vi "KeySwitched.vi"(8 "error in (no error)":errorcluster, 9 "Key":T1 {"Time" format="%<%.3X>T"}, 11 "Gviewer in":refnum<class "Gviewer.lvclass">) -> (0 "error out":errorcluster, 3 "Gviewer out":refnum<class "Gviewer.lvclass">, 5 "Char":i16)   [LabVIEW 2020, in "Sgraph_lib_V1.lvlib" / "Gviewer.lvclass"]
doc: "Andre Koelewijn, 8 jan 2021\n\nIf a switch is pressed then this VI hold the code for the action.\nIf a key stroke combined with another action is used then it is possible that such code resides in another part of the program."
uses:
  Gviewer.lvclass
  controls/KeyPress.ctl
  <vilib>/event_ctls.llb/eventvkey.ctl
  Gviewer.lvclass/Gviewer.ctl
  Common/controls/ToolTypeEnum.ctl
  Builds/Sgraph_lib_V1.lvlib
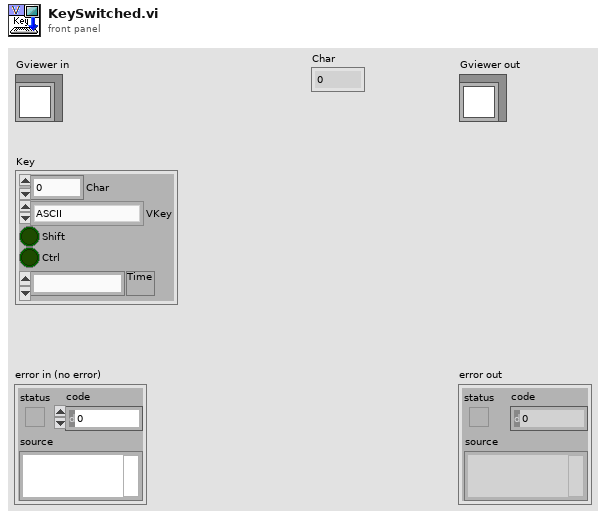
[diagram p1: front panel]
types:
  T1 = typedef "Sgraph_lib_V1.lvlib/Gviewer.lvclass/KeyPress.ctl" = cluster{"Char":i16, "VKey":T2, "Shift":bool, "Ctrl":bool, "Time":timestamp}
  T2 = typedef "eventvkey.ctl" = enum16{"ASCII", "Enter", "Return", "Shift", "Ctrl", "Alt", "Cmd", "Opt", "Caps", "NumLock", "Clear", "Break", "Up", "Down", "Left", "Right", "Insert", "Delete", "Home", "End", "PageUp", "PageDown", "Escape", "Help", "Pause", "ScrollLock", "F1", "F2", "F3", "F4", "F5", "F6", "F7", "F8", "F9", "F10", "F11", "F12", "F13", "F14", "F15", "F16", "F17", "F18", "F19", "F20", "F21", "F22", "F23", "F24", "Play", "VolumeUp", "VolumeDown", "Mute", "Two Byte Char"}
  T3 = typedef "Sgraph_lib_V1.lvlib/ToolTypeEnum.ctl" = enum16{"00_Esc button", "01_Undo", "02_HelpButton", "03_CursorViewButton", "04_AutoScale_Fit", "05_AutoScale_Stacked", "06_ZoomWindowStart", "07_ZoomTimeStart", "08_ZoomAmplitudeStart", "09", "10", "11", "12", "13", "14", "15", "16", "17", "18", "19", "20_VerticalScroll", "21_VerticalMove", "22_TimeScroll", "23_TimeMove", "24", "25", "26_ZoomWindowSize", "27_ZoomTimeWindowSize", "28_ZoomAmplitudeWindowSize", "29", "30_LegendMovePoint", "31_LegendMoveDrag", "32", "33", "34", "35", "36", "37", "38", "39", "40_AddYscalePoint", "41_AddYscalePlace", "42_AddYscaleMovePoint", "43_AddYscaleMoveDrag", "44_AddYscaleDeletePoint"}
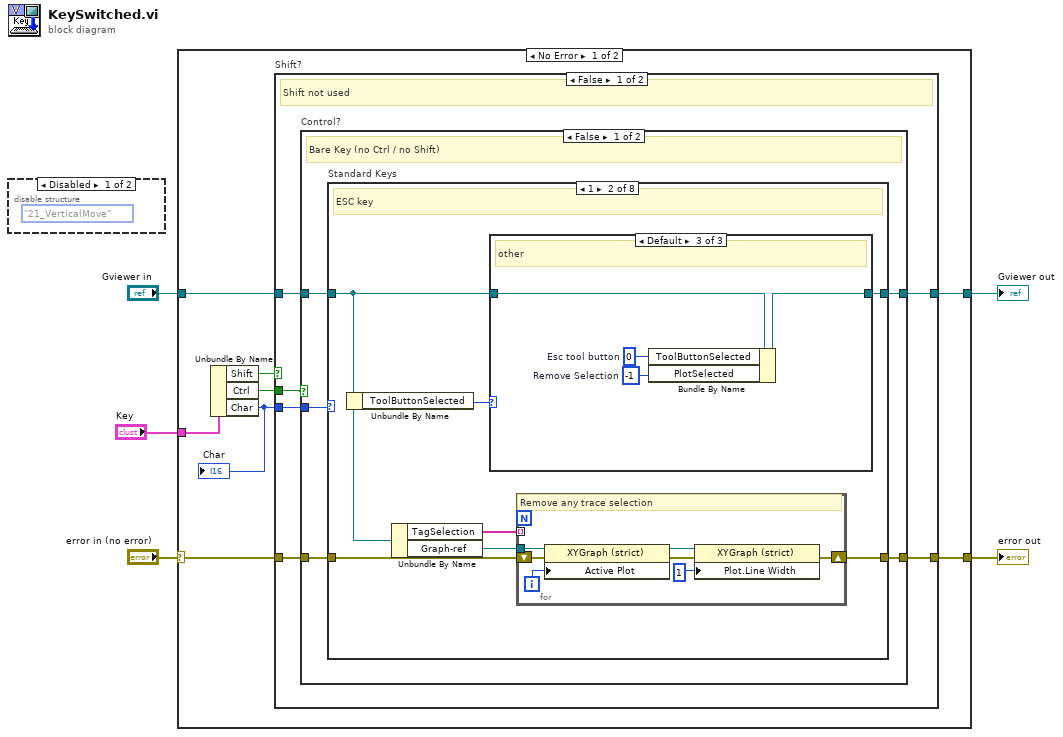
[diagram p0: block diagram]
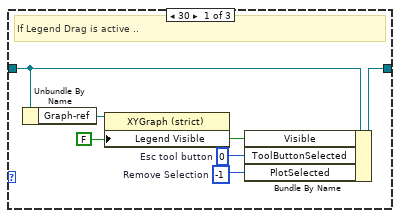
[diagram p4: hidden frame]
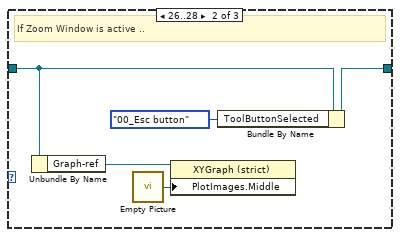
[diagram p5: hidden frame]
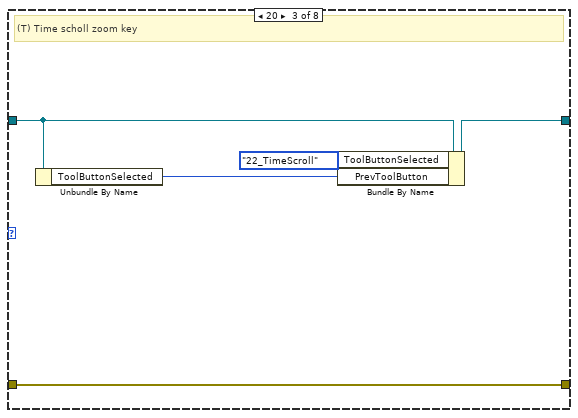
[diagram p6: hidden frame]
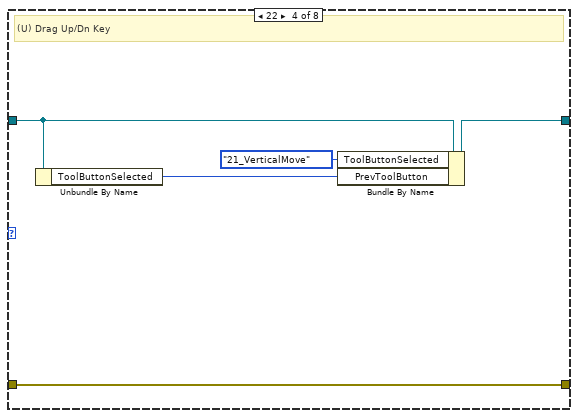
[diagram p7: hidden frame]
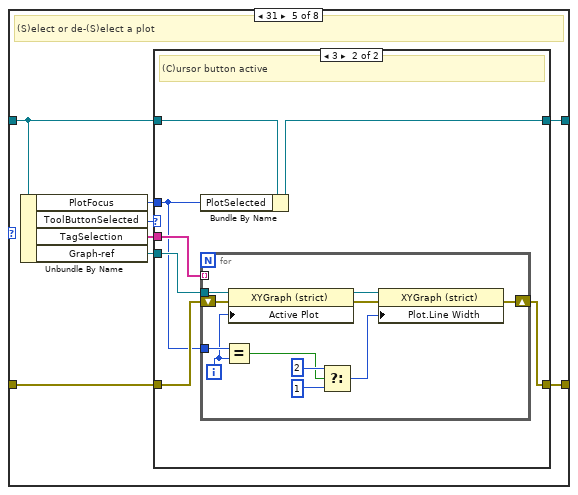
[diagram p8: hidden frame]
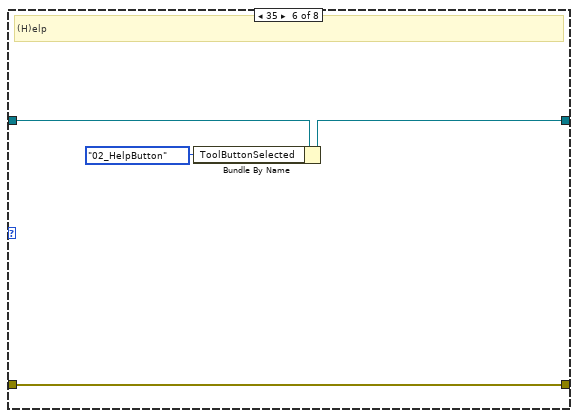
[diagram p10: hidden frame]
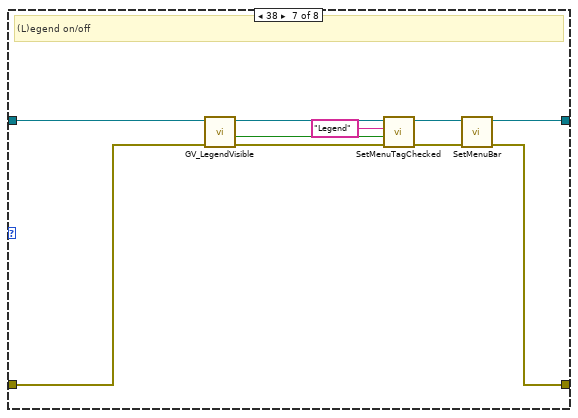
[diagram p11: hidden frame]
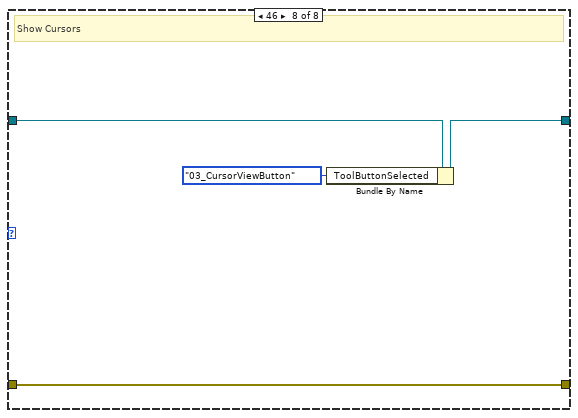
[diagram p12: hidden frame]
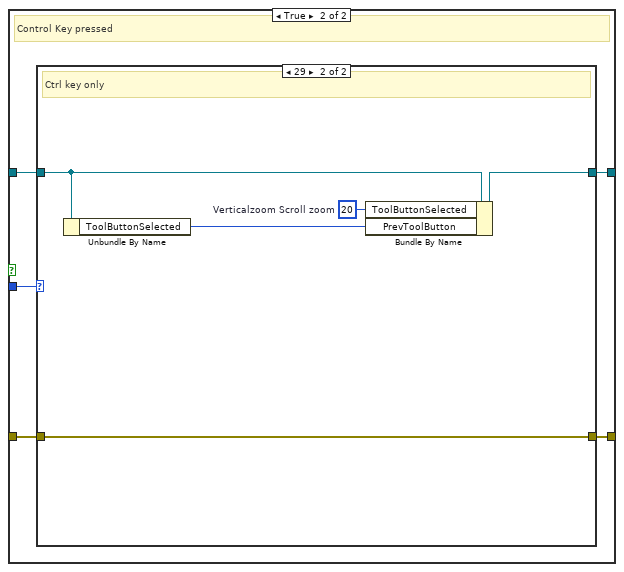
[diagram p13: hidden frame]
diagram:
  n1 = disable-structure shown="Disabled" {
    frame Disabled {
      (unwired) ToolTypeEnum."21_VerticalMove" ("Enum")
    }
    frame Enabled {
    }
  }
  n2 = case shown="No Error" "error in (no error)" {
    selector: "error in (no error)" -> [w8 w134]
    tunnel: [w7 w134] -> w4
    tunnel: [w9 w133] -> w2
    tunnel: "Gviewer in" -> [w10 w133]
    tunnel: "Key" -> [w13 _]
    frame No Error {
      n3 = Unbundle By Name(w13) -> ("Shift"=w12:bool, "Ctrl"=w11:bool, "Char"=w6:i16)
      "Char" <- w6
      n4 = case "Shift?" shown="False" w12 {
        tunnel: w11 -> [w19 w128]
        tunnel: w10 -> [w18 w127]
        tunnel: [w17 w126] -> w9
        tunnel: w8 -> [w16 w125]
        tunnel: [w15 w124] -> w7
        tunnel: w6 -> [w14 _]
        frame False {
          # "Shift not used"
          n5 = case "Control?" shown="False" w19 {
            tunnel: [w22 w114] -> w17
            tunnel: w18 -> [w23 w115]
            tunnel: [w20 w112] -> w15
            tunnel: w16 -> [w21 w113]
            tunnel: w14 -> [w24 w116]
            frame False {
              # "Bare Key (no Ctrl / no Shift)"
              n6 = case "Standard Keys" shown="1" w24 {
                tunnel: w23 -> [w26 w28 w59 w64 w70 w95 w101 w109]
                tunnel: [w26 w33 w58 w63 w69 w96 w104 w110] -> w22
                tunnel: [w25 w30 w57 w62 w72 w97 w103 w111] -> w20
                tunnel: w21 -> [w25 w29 w57 w62 w73 w97 w100 w111]
                frame Default {
                  # "Not implemented"
                }
                frame 1 {
                  # "ESC key"
                  n7 = Unbundle By Name(w28) -> ("ToolButtonSelected"=w27:i32)
                  n8 = Unbundle By Name(w28) -> ("TagSelection"=w32:string[], "Graph-ref"=w31:refnum<vi>)
                  n9 = case shown="Default" w27 {
                    tunnel: [w39 w44 w47] -> w33
                    tunnel: w28 -> [w36 w43 w45]
                    frame 30 {
                      w34 = -1  # Remove Selection
                      w35 = 0  # Esc tool button
                      w37 = FALSE
                      # "If Legend Drag is active .."
                      n10 = Unbundle By Name(w36) -> ("Graph-ref"=w38:refnum<vi>)
                      n11 = property class="XYGraph (strict)"(reference=w38, "Legend Visible"=w37) -> ()  [unwired: 1 in, 2 out]
                      n12 = Bundle By Name(cluster=w36, "Visible"=w37, "ToolButtonSelected"=w35, "PlotSelected"=w34) -> (w39:refnum<class "Gviewer.lvclass">)
                    }
                    frame 26..28 {
                      # "If Zoom Window is active .."
                      n13 = Unbundle By Name(w43) -> ("Graph-ref"=w41:refnum<vi>)
                      n14 = call "Empty Picture"() -> ("empty picture"=w42:picture)
                      n15 = property class="XYGraph (strict)"(reference=w41, "PlotImages.Middle"=w42) -> ()  [unwired: 1 in, 2 out]
                      n16 = Bundle By Name(cluster=w43, "ToolButtonSelected"=ToolTypeEnum."00_Esc button" ("Enum")) -> (w44:refnum<class "Gviewer.lvclass">)
                    }
                    frame Default {
                      w46 = -1  # Remove Selection
                      w48 = 0  # Esc tool button
                      # "other"
                      n17 = Bundle By Name(cluster=w45, "ToolButtonSelected"=w48, "PlotSelected"=w46) -> (w47:refnum<class "Gviewer.lvclass">)
                    }
                  }
                  n18 = for {
                    tunnel: w31 -> [w55]
                    shift-right: [w51] -> w30
                    shift-left: w29 -> [w53]
                    tunnel: w32 -> [_] mode=indexing
                    i -> [w50]
                    # "Remove any trace selection"
                    n19 = property class="XYGraph (strict)"(reference=w55, error in=w53, "Active Plot"=w50) -> (reference out=w54:refnum<vi>, error out=w52:errorcluster)
                    n20 = property class="XYGraph (strict)"(reference=w54, error in=w52, "Plot.Line Width"=u8 1) -> (error out=w51:errorcluster)  [unwired: 1 out]
                  }
                }
                frame 20 {
                  # "(T) Time scholl zoom key"
                  n21 = Unbundle By Name(w59) -> ("ToolButtonSelected"=w60:i32)
                  n22 = Bundle By Name(cluster=w59, "ToolButtonSelected"=ToolTypeEnum."22_TimeScroll" ("Enum"), "PrevToolButton"=w60) -> (w58:refnum<class "Gviewer.lvclass">)
                }
                frame 22 {
                  # "(U) Drag Up/Dn Key"
                  n23 = Unbundle By Name(w64) -> ("ToolButtonSelected"=w65:i32)
                  n24 = Bundle By Name(cluster=w64, "ToolButtonSelected"=ToolTypeEnum."21_VerticalMove" ("Enum"), "PrevToolButton"=w65) -> (w63:refnum<class "Gviewer.lvclass">)
                }
                frame 31 {
                  # "(S)elect or de-(S)elect a plot"
                  n25 = Unbundle By Name(w70) -> ("PlotFocus"=w68:i32, "ToolButtonSelected"=w71:i32, "TagSelection"=w67:string[], "Graph-ref"=w66:refnum<vi>)
                  n26 = case shown="3" w71 {
                    tunnel: w73 -> [w74 w79]
                    tunnel: [w74 w78] -> w72
                    tunnel: w70 -> [w75 w81]
                    tunnel: [w75 w82] -> w69
                    tunnel: w68 -> [_ w76]
                    tunnel: w67 -> [_ w80]
                    tunnel: w66 -> [_ w77]
                    frame Default {
                    }
                    frame 3 {
                      # "(C)ursor button active"
                      n27 = Bundle By Name(cluster=w81, "PlotSelected"=w76) -> (w82:refnum<class "Gviewer.lvclass">)
                      n28 = for {
                        tunnel: w80 -> [_] mode=indexing
                        tunnel: w76 -> [w85]
                        tunnel: w77 -> [w93]
                        shift-right: [w87] -> w78
                        shift-left: w79 -> [w89]
                        i -> [w84]
                        n29 = Equal?(x=w85, y=w84) -> (x = y?=w86:bool)
                        n30 = property class="XYGraph (strict)"(reference=w93, error in=w89, "Active Plot"=w84) -> (reference out=w92:refnum<vi>, error out=w88:errorcluster)
                        n31 = Select(t=u8 2 ("Plot.Line Width"), s=w86, f=u8 1 ("Plot.Line Width")) -> (s? t:f=w90:u8)
                        n32 = property class="XYGraph (strict)"(reference=w92, error in=w88, "Plot.Line Width"=w90) -> (error out=w87:errorcluster)  [unwired: 1 out]
                      }
                    }
                  }
                }
                frame 35 {
                  # "(H)elp"
                  n33 = Bundle By Name(cluster=w95, "ToolButtonSelected"=ToolTypeEnum."02_HelpButton" ("Enum")) -> (w96:refnum<class "Gviewer.lvclass">)
                }
                frame 38 {
                  # "(L)egend on/off"
                  n34 = call "GV_LegendVisible.vi"("error in (no error)"=w100, "Gviewer in"=w101) -> ("error out"=w99:errorcluster, "Visible?"=w98:bool, "Gviewer out"=w102:refnum<class "Gviewer.lvclass">)  [unwired: 7 in]
                  n35 = call "SetMenuTagChecked.vi"("error in (no error)"=w99, "Checked"=w98, "TAG"="Legend", "Gviewer in"=w102) -> ("error out"=w107:errorcluster, "Gviewer out"=w106:refnum<class "Gviewer.lvclass">)  [unwired: 6 in]
                  n36 = call "SetMenuBar.vi"("error in (no error)"=w107, "Gviewer in"=w106) -> ("error out"=w103:errorcluster, "Gviewer out"=w104:refnum<class "Gviewer.lvclass">)  [unwired: 8 in]
                }
                frame 46 {
                  # "Show Cursors"
                  n37 = Bundle By Name(cluster=w109, "ToolButtonSelected"=ToolTypeEnum."03_CursorViewButton" ("Enum")) -> (w110:refnum<class "Gviewer.lvclass">)
                }
              }
            }
            frame True {
              # "Control Key pressed"
              n38 = case shown="29" w116 {
                tunnel: w115 -> [w118 w120]
                tunnel: [w118 w121] -> w114
                tunnel: w113 -> [w117 w123]
                tunnel: [w117 w123] -> w112
                frame Default {
                  # "Not defined"
                }
                frame 29 {
                  w122 = 20  # Verticalzoom Scroll zoom
                  # "Ctrl key only"
                  n39 = Unbundle By Name(w120) -> ("ToolButtonSelected"=w119:i32)
                  n40 = Bundle By Name(cluster=w120, "ToolButtonSelected"=w122, "PrevToolButton"=w119) -> (w121:refnum<class "Gviewer.lvclass">)
                }
              }
            }
          }
        }
        frame True {
          # "Shift Pressed"
          n41 = case "Control?" shown="False" w128 {
            tunnel: w127 -> [w130 w132]
            tunnel: [w130 w132] -> w126
            tunnel: w125 -> [w129 w131]
            tunnel: [w129 w131] -> w124
            frame False {
              # "Control Key not pressed: Only Shift Key used"
            }
            frame True {
              # "Control Key Pressed"
            }
          }
        }
      }
    }
    frame Error {
    }
  }
  "error out" <- w4
  "Gviewer out" <- w2
